vi "Create Section Cluster.vi"(8 "error in":errorcluster, 9 "Node Clusters":refnum<vi>[](array[refnum]), 10 "Node Types":string[](array[string]), 11 "Sections":refnum<k20>[](array[refnum])) -> (0 "error out":errorcluster, 1 "Node Clusters":refnum<vi>[](array[refnum]), 2 "Node Types":string[](array[string]), 3 "Sections":refnum<k20>[](array[refnum]))   [LabVIEW 2026, in "XML Parser.lvlib"]
uses:
  XML Parser.lvlib
  <resource>/objmgr/DOMUserDefRef.rc
  <vilib>/xml/NI_XML.lvlib
  <vilib>/Utility/miscctls.llb/LVPositionTypeDef.ctl
  <vilib>/xml/Close Reference(Node).vi
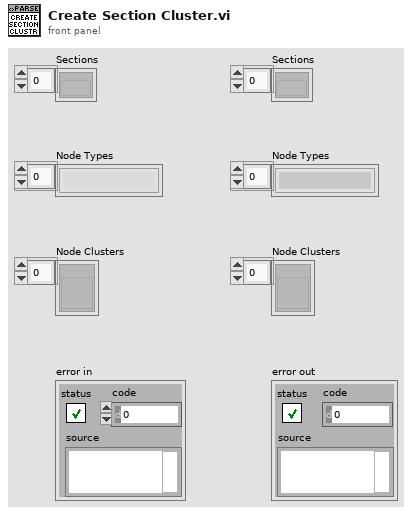
[diagram p1: front panel]
types:
  T1 = typedef "LVPositionTypeDef.ctl" = cluster{"Left":i32, "Top":i32}
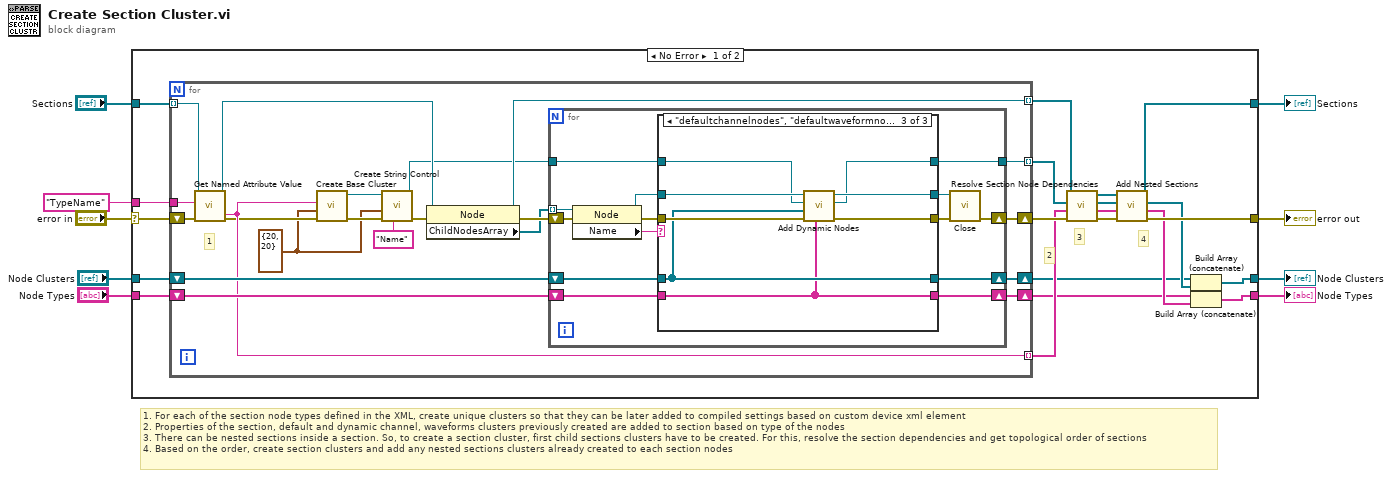
[diagram p0: block diagram]
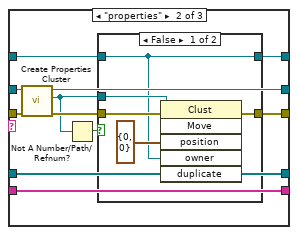
[diagram p3: hidden frame]
diagram:
  # "1. For each of the section node types defined in the XML, create unique clusters so that they can be later added to compiled settings based on custom device xml element\n2. Properties of the section, default and dynamic channel, waveforms clusters previously created are added to section based on type of the nodes\n3. There can be nested sections inside a section. So, to create a section cluster, first child sections clusters have to be created. For this, resolve the section dependencies and get topological order of sections\n4. Based on the order, create section clusters and add any nested sections clusters already created to each section nodes"
  n1 = case shown="No Error" "error in" {
    selector: "error in" -> [w29 w100]
    tunnel: [w30 w100] -> w8
    tunnel: "Sections" -> [w21 w97]
    tunnel: "Node Types" -> [w11 w99]
    tunnel: "Node Clusters" -> [w14 w98]
    tunnel: [w24 w99] -> w4
    tunnel: [w22 w98] -> w3
    tunnel: [w26 w97] -> w2
    tunnel: "TypeName" ("Attribute Name") -> [w10 _]
    frame No Error {
      # "4"
      # "3"
      # "2"
      n2 = for {
        tunnel: w21 -> [w47] mode=indexing
        shift-right: [w51] -> w28
        shift-left: w29 -> [w49]
        tunnel: [w41] -> w16 mode=indexing
        tunnel: [w43] -> w18 mode=indexing
        tunnel: [w42] -> w20 mode=indexing
        shift-right: [w33] -> w13
        shift-left: w14 -> [w44]
        shift-right: [w32] -> w12
        shift-left: w11 -> [w45]
        tunnel: w10 -> [w31]
        w36 = cluster{"Horizontal":i16, "Vertical":i16} {"Horizontal"=20, "Vertical"=20} ("Point")
        # "1"
        n3 = call "Get Named Attribute Value.vi"("error in"=w49, "Attribute Name"=w31, "Node In"=w47) -> ("error out"=w40:errorcluster, "Node Out"=w46:refnum<k20>, "Attribute Value"=w41:string)  [unwired: 5 in, 1 out]
        n4 = call "Create Base Cluster.vi"("error in"=w40, "Location"=w36, "Cluster Name"=w41) -> ("error out"=w39:errorcluster, "Cluster out"=w35:refnum<vi>)  [unwired: 6 in, 1 out]
        n5 = call "Create String Control.vi"("Label.Text"="Name", "error in"=w39, "location"=w36, "Cluster in"=w35) -> ("error out"=w38:errorcluster, "Cluster out"=w34:refnum<vi>)  [unwired: 6 in]
        n6 = property class="Node"(reference=w46, error in=w38) -> (reference out=w42:refnum<k20>, error out=w50:errorcluster, "ChildNodesArray"=w48:refnum<k20>[])
        n7 = for {
          tunnel: w48 -> [w61] mode=indexing
          shift-right: [w64] -> w51
          shift-left: w50 -> [w65]
          tunnel: w34 -> [w57]
          tunnel: [w54] -> w43
          shift-right: [w53] -> w33
          shift-left: w44 -> [w55]
          shift-right: [w52] -> w32
          shift-left: w45 -> [w56]
          n8 = property class="Node"(reference=w61, error in=w65) -> (reference out=w59:refnum<k20>, error out=w63:errorcluster, "Name"=w60:string)
          n9 = case shown="\"defaultchannelnodes\", \"defaultwaveformnodes\", \"dynamicchannelnodes\", \"dynamicwaveformnodes\"" w60 {
            tunnel: w59 -> [w69 w78 w94]
            tunnel: [w69 w77 w92] -> w58
            tunnel: w57 -> [w68 w76 w93]
            tunnel: w63 -> [w70 w81 w96]
            tunnel: [w70 w79 w95] -> w62
            tunnel: [w68 w73 w91] -> w54
            tunnel: w56 -> [w66 w71 w89]
            tunnel: w55 -> [w67 w72 w90]
            tunnel: [w67 w72 w90] -> w53
            tunnel: [w66 w71 w89] -> w52
            frame Default {
            }
            frame "properties" {
              n10 = call "Create Properties Cluster.vi"("error in"=w81, "Node In"=w78) -> ("error out"=w80:errorcluster, "Clust Refnum"=w74:refnum<vi>, "Node Out"=w77:refnum<k20>)  [unwired: 7 in]
              n11 = Not A Number/Path/Refnum?(number/path/refnum=w74) -> (NaN/Path/Refnum?=w75:bool)
              n12 = case shown="False" w75 {
                tunnel: w76 -> [w82 w87]
                tunnel: w80 -> [w86 w88]
                tunnel: [w85 w88] -> w79
                tunnel: w74 -> [w83 _]
                tunnel: [w82 w87] -> w73
                frame False {
                  n13 = invoke class="Clust" method="Move"(reference=w83, error in=w86, "position"=T1 {"Left"=0, "Top"=0}, "owner"=w82) -> (error out=w85:errorcluster)  [unwired: 2 in, 5 out]
                }
                frame True {
                }
              }
            }
            frame "defaultchannelnodes", "defaultwaveformnodes", "dynamicchannelnodes", "dynamicwaveformnodes" {
              n14 = call "Add Dynamic Nodes.vi"("Node Types"=w89, "error in"=w96, "Node Clusters"=w90, "Clust Refnum"=w93, "Node"=w94) -> ("error out"=w95:errorcluster, "Clust Refnum"=w91:refnum<vi>, "Node"=w92:refnum<k20>)  [unwired: 2 in, 2 out]
            }
          }
          n15 = call-poly <vilib>:"Close.vi"("error in (no error)"=w62, "node"=w58) -> ("error out"=w64:errorcluster)  [unwired: 7 in]
        }
      }
      n16 = call "Resolve Section Node Dependencies.vi"("error in"=w28, "Section Types"=w16, "Section Clusters"=w18, "Sections"=w20) -> ("error out"=w27:errorcluster, "Section Types"=w15:string[], "Section Clusters"=w17:refnum<vi>[], "Sections"=w19:refnum<k20>[])  [unwired: 4 in]
      n17 = call "Add Nested Sections.vi"("error in"=w27, "Section Types"=w15, "Section Clusters"=w17, "Sections"=w19) -> ("error out"=w30:errorcluster, "Section Types"=w25:string[], "Section Clusters"=w23:refnum<vi>[], "Sections"=w26:refnum<k20>[])  [unwired: 4 in]
      n18 = Build Array (concatenate)(w13, w23) -> (w22:refnum<vi>[])
      n19 = Build Array (concatenate)(w12, w25) -> (w24:string[])
    }
    frame Error {
    }
  }
  "error out" <- w8
  "Node Types" <- w4
  "Node Clusters" <- w3
  "Sections" <- w2
